vi "Model Initial Values - Model On Load Action.vi"(8 "error in (no error)":errorcluster, 11 "Device Item Ref in":T1 format="%.0x") -> (0 "error out":errorcluster, 3 "Device Item Ref out":T1 format="%.0x")   [LabVIEW 2011, in "Model Initial Values Custom Device.lvlib"]
uses:
  Model Initial Values Custom Device.lvlib
  <vilib>/NI Veristand/Custom Device API/Custom Device Item Ref.ctl
  Model Initial Values - Global.vi
  <vilib>/NI Veristand/Custom Device API/Custom Device API.lvlib
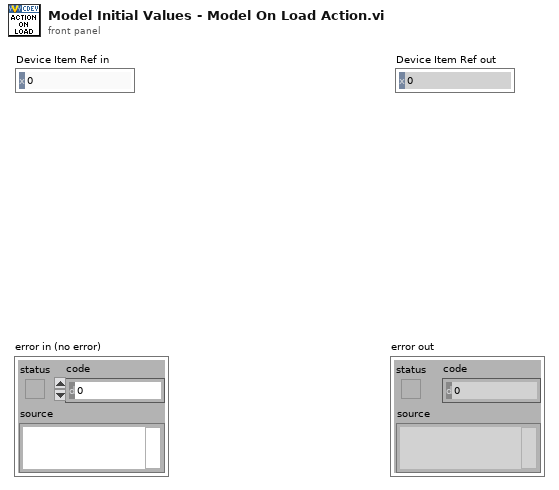
[diagram p1: front panel]
types:
  T1 = typedef "Custom Device API.lvlib/Custom Device Item Ref.ctl" = u64
  T2 = enum16{"Open or Add", "Close Ref", "Reset Local Store"}
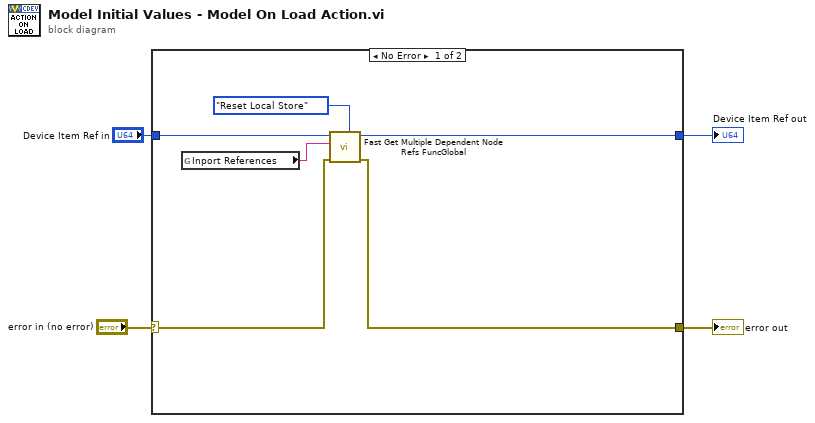
[diagram p0: block diagram]
diagram:
  n1 = case shown="No Error" "error in (no error)" {
    selector: "error in (no error)" -> [w6 w12]
    tunnel: [w5 w12] -> w3
    tunnel: "Device Item Ref in" -> [w10 w11]
    tunnel: [w9 w11] -> w1
    frame No Error {
      n2 = global read "Model Initial Values - Global.vi" "Inport References"() -> (w7:string)
      n3 = call "Fast Get Multiple Dependent Node Refs FuncGlobal.vi"("Action"=T2."Reset Local Store", "error in (no error)"=w6, "Base Property Name"=w7, "Item Ref in"=w10) -> ("error out"=w5:errorcluster, "Item Ref out"=w9:T1)  [unwired: 5 in, 1 out]
    }
    frame Error {
    }
  }
  "error out" <- w3
  "Device Item Ref out" <- w1
